vi "PathPlanner_Path_GetGlobalConstraints.vi"(11 "PathPlannerPath":T2={"BezierPoints"=[], "PreviewStartingRotation"={"VALUE"=0.0, "COS"=1.0, "SIN"=0.0}, "Reversed"=FALSE, "RotationTargets"=[], "ConstraintZones"=[], "EventMarkers"=[], "GlobalConstraints"={"MaxVelocityMps;"=0.0, "MaxAccelerationMpsSq;"=0.0, "MaxAngularVelRadPsEc;"=0.0, "MaxAngularAccRadPSecSq"=0.0, "Exists"=FALSE}, "GoalEndState"={"Velocity"=0.0, "Rotation"={"VALUE"=0.0, "COS"=1.0, "SIN"=0.0}}, "AllPoints"=[]} {"AllPoints"."HolonomicRotation"."SIN" format="%13.4f"; "AllPoints"."HolonomicRotation"."COS" format="%13.4f"; "AllPoints"."HolonomicRotation"."VALUE" format="%13.4f"; "AllPoints"."Position"."Y" format="%14.3f"; "AllPoints"."Position"."X" format="%14.3f"; "GoalEndState"."Rotation"."SIN" format="%13.4f"; "GoalEndState"."Rotation"."COS" format="%13.4f"; "GoalEndState"."Rotation"."VALUE" format="%13.4f"; "EventMarkers"."lastRobotPos"."Y" format="%14.3f"; "EventMarkers"."lastRobotPos"."X" format="%14.3f"; "EventMarkers"."markerPos"."Y" format="%14.3f"; "EventMarkers"."markerPos"."X" format="%14.3f"; "RotationTargets"."target"."SIN" format="%13.4f"; "RotationTargets"."target"."COS" format="%13.4f"; "RotationTargets"."target"."VALUE" format="%13.4f"; "PreviewStartingRotation"."SIN" format="%13.4f"; "PreviewStartingRotation"."COS" format="%13.4f"; "PreviewStartingRotation"."VALUE" format="%13.4f"; "BezierPoints"."Y" format="%14.3f"; "BezierPoints"."X" format="%14.3f"}) -> (3 "GlobalConstraints":T1)   [LabVIEW 2019, in "PathPlanner24.lvlib"]
doc: "Get the global constraints for this path\n \nInputs: \n - Path - cluster - path definition data structure\n\nOutputs:\n - GlobalConstraints - cluster - Global constraints that apply to this path"
uses:
  PathPlanner24.lvlib
  TypeDef/PathPlannerPath.ctl
  <vilib>/Rock Robotics/WPI/ThirdParty/JAS_Junk/TrajLib/TypeDef/TRANSLATION2D.ctl
  <vilib>/Rock Robotics/WPI/ThirdParty/JAS_Junk/TrajLib/TypeDef/ROTATION2D.ctl
  TypeDef/PathPlannerRotationTarget.ctl
  TypeDef/PathPlannerConstraintsZone.ctl
  TypeDef/PathPlannerPathConstraints.ctl
  TypeDef/PathPlannerEventMarker.ctl
  TypeDef/PathPlannerCommandUtil.ctl
  ENum/PathPlanner_CommandUtilType_ENUM.ctl
  TypeDef/PathPlannerGoalEndState.ctl
  TypeDef/PathPlannerPathPoint.ctl
  <vilib>/Rock Robotics/WPI/ThirdParty/JAS_Junk/TrajLib/Trajectory_Library.lvlib
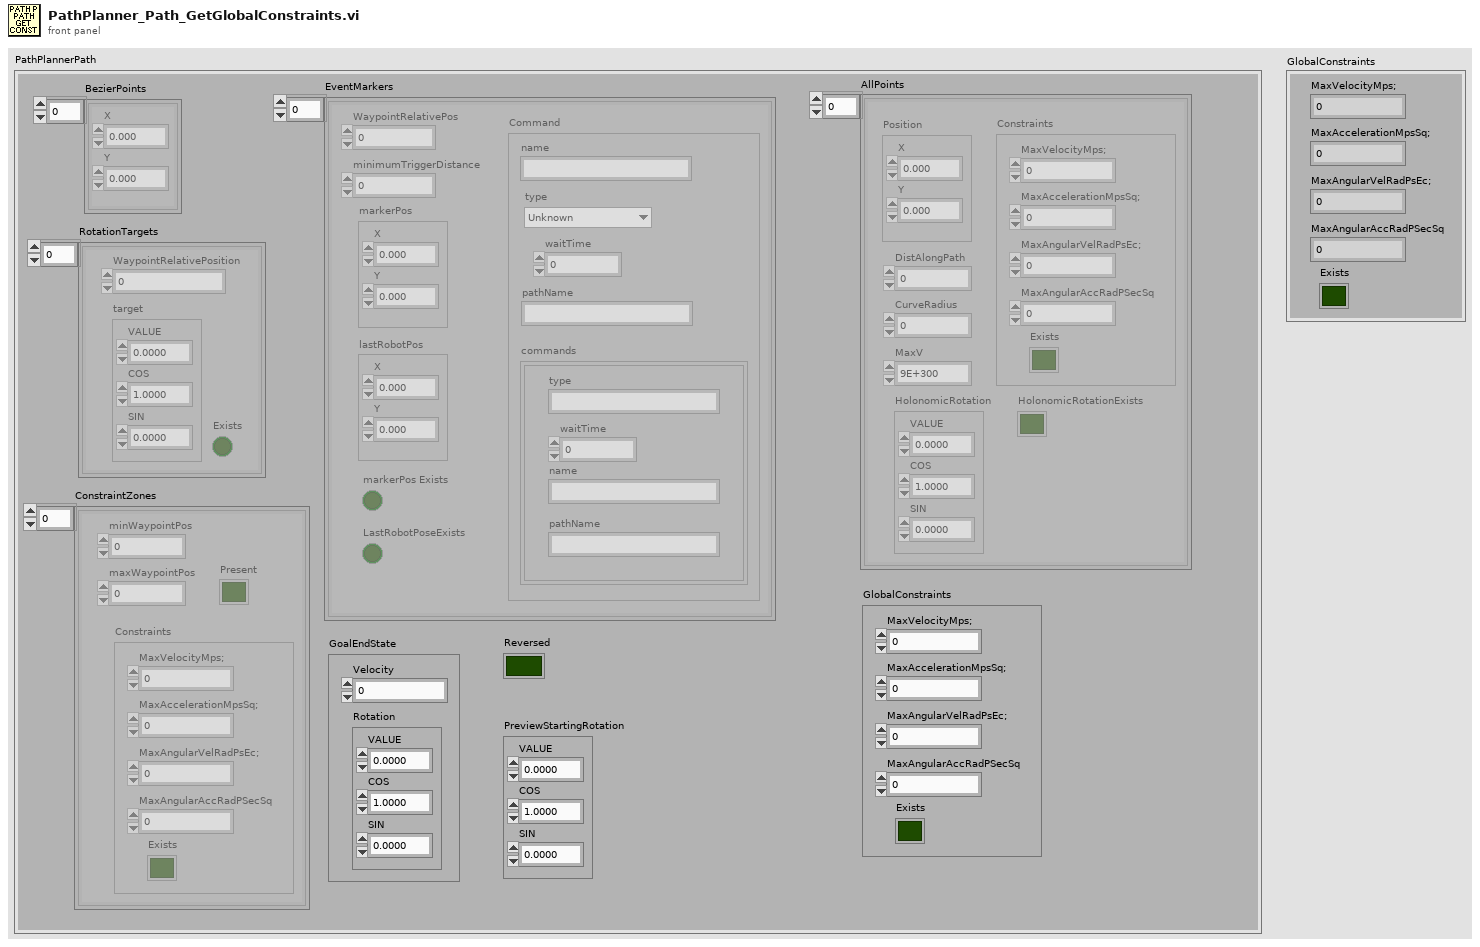
[diagram p1: front panel]
types:
  T1 = typedef "PathPlanner24.lvlib/PathPlannerPathConstraints.ctl" = cluster{"MaxVelocityMps;":dbl, "MaxAccelerationMpsSq;":dbl, "MaxAngularVelRadPsEc;":dbl, "MaxAngularAccRadPSecSq":dbl, "Exists":bool}
  T2 = typedef "PathPlanner24.lvlib/PathPlannerPath.ctl" = cluster{"BezierPoints":T3[], "PreviewStartingRotation":T4, "Reversed":bool, "RotationTargets":T5[], "ConstraintZones":T6[], "EventMarkers":T7[], "GlobalConstraints":T1, "GoalEndState":T10, "AllPoints":T11[]}
  T3 = typedef "Trajectory_Library.lvlib/TRANSLATION2D.ctl" = cluster{"X":dbl, "Y":dbl}
  T4 = typedef "Trajectory_Library.lvlib/ROTATION2D.ctl" = cluster{"VALUE":dbl, "COS":dbl, "SIN":dbl}
  T5 = typedef "PathPlanner24.lvlib/PathPlannerRotationTarget.ctl" = cluster{"target":T4, "WaypointRelativePosition":dbl, "Exists":bool}
  T6 = typedef "PathPlanner24.lvlib/PathPlannerConstraintsZone.ctl" = cluster{"minWaypointPos":dbl, "maxWaypointPos":dbl, "Constraints":T1, "Present":bool}
  T7 = typedef "PathPlanner24.lvlib/PathPlannerEventMarker.ctl" = cluster{"WaypointRelativePos":dbl, "minimumTriggerDistance":dbl, "markerPos":T3, "lastRobotPos":T3, "Command":T8, "markerPos Exists":bool, "LastRobotPoseExists":bool}
  T8 = typedef "PathPlanner24.lvlib/PathPlannerCommandUtil.ctl" = cluster{"waitTime":dbl, "name":string, "pathName":string, "commands":cluster{"type":string, "waitTime":dbl, "name":string, "pathName":string}[], "type":T9}
  T9 = typedef "PathPlanner24.lvlib/PathPlanner_CommandUtilType_ENUM.ctl" = enum16{"Unknown", "Wait", "Named", "Path", "Sequential", "Parallel", "Race", "Deadline"}
  T10 = typedef "PathPlanner24.lvlib/PathPlannerGoalEndState.ctl" = cluster{"Velocity":dbl, "Rotation":T4}
  T11 = typedef "PathPlanner24.lvlib/PathPlannerPathPoint.ctl" = cluster{"Position":T3, "HolonomicRotation":T4, "DistAlongPath":dbl, "CurveRadius":dbl, "MaxV":dbl, "Constraints":T1, "HolonomicRotationExists":bool}
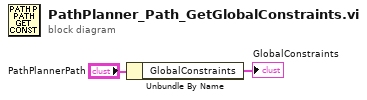
[diagram p0: block diagram]
diagram:
  n1 = Unbundle By Name("PathPlannerPath") -> ("GlobalConstraints"=→"GlobalConstraints":T1)
